vi "GetAndLockBuffers.vi"(7 "names":string[](array[string]), 8 "error in":errorcluster, 9 "ms timeout (-1)":i32=-1, 10 "size":u64, 11 "amount of buffers":u16) -> (0 "error out":errorcluster, 2 "ptrs":u64[](array[numeric]))   [LabVIEW 2016]
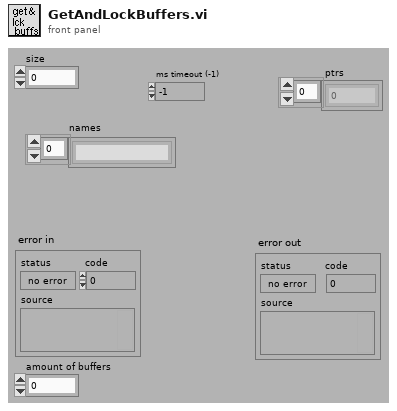
[diagram p1: front panel]
types:
  T1 = cluster{"Name":string, "size (bytes)":u64, "pointer":u64, "Lock":bool}
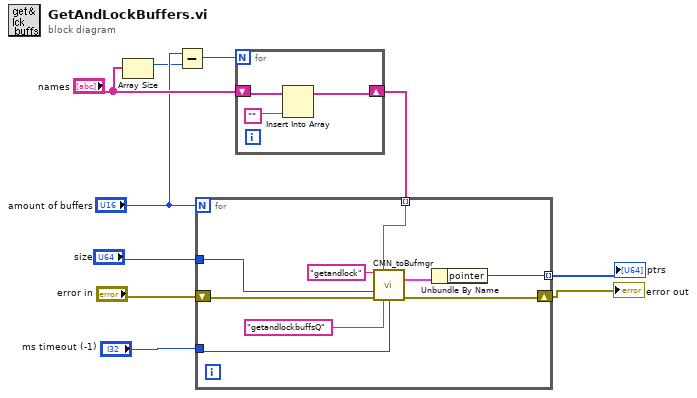
[diagram p0: block diagram]
diagram:
  n1 = Array Size(array="names") -> (size(s)=w3:i32)
  n2 = Subtract(x="amount of buffers", y=w3) -> (x-y=w2:i32)
  n3 = for {
    N: w2 -> [_]
    shift-right: [w11] -> w1
    shift-left: "names" -> [w13]
    n4 = Insert Into Array(array=w13, new element="") -> (w11:string[])  [unwired: 1 in]
  }
  n5 = for {
    N: "amount of buffers" -> [_]
    shift-right: [w21] -> w8
    shift-left: "error in" -> [w22]
    tunnel: "ms timeout (-1)" -> [w20]
    tunnel: "size" -> [w18]
    tunnel: [w16] -> w7 mode=indexing
    tunnel: w1 -> [w14] mode=indexing
    n6 = call "CMN_toBufmgr.vi"("command"="getandlock", "bufname"=w14, "bufsize"=w18, "error in"=w22, "responseQ"="getandlockbuffsQ", "ms timeout (-1)"=w20) -> ("buffer"=w17:T1, "error out"=w21:errorcluster)  [unwired: 2 in, 6 out]
    n7 = Unbundle By Name(w17) -> ("pointer"=w16:u64)
  }
  "error out" <- w8
  "ptrs" <- w7
